vi "sub_USRP_init_Rx.vi"(11 "Rx Parameters":T1={"IQ rate (Hz)"=200000.0, "Carrier frequency [Hz]"=1187500000.0, "Gain [dB]"=16.0, "Antenna"="RX1", "Rx device name"="192.168.10.4; 192.168.10.5;"} {"Gain [dB]" format="%#_6f"; "Carrier frequency [Hz]" format="%#_6p"; "IQ rate (Hz)" format="%#_6p"}) -> (0 "Error out":errorcluster, 3 "Rx Session handle out":refnum<k15>="192.168.10.3 (5)")   [LabVIEW 2012]
uses:
  <instrlib>/niUSRP/niUSRP Timestamp.ctl
  <instrlib>/niUSRP/niUSRP Configure Time Start Trigger.vi
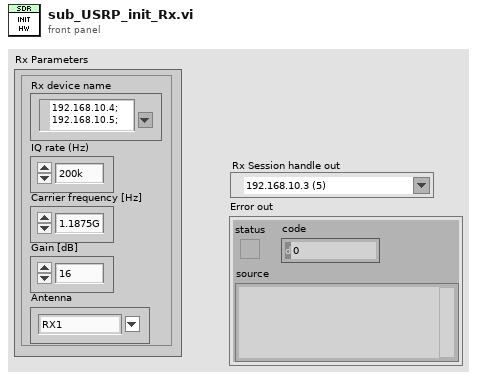
[diagram p1: front panel]
types:
  T1 = cluster{"IQ rate (Hz)":dbl, "Carrier frequency [Hz]":dbl, "Gain [dB]":dbl, "Antenna":string, "Rx device name":refnum<k15>}
  T2 = typedef "niUSRP Timestamp.ctl" = cluster{"whole seconds":u64, "fractional seconds":dbl}
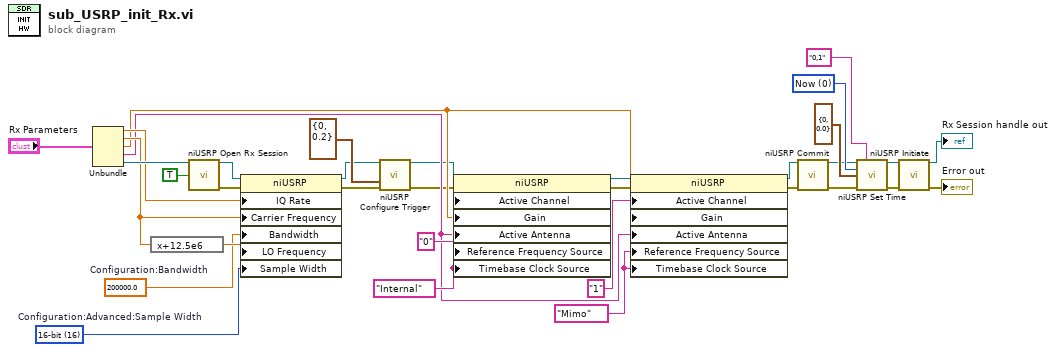
[diagram p0: block diagram]
diagram:
  w7 = 0 items=["Now", "Next Timebase Edge"] ("apply timestamp")
  w22 = "Mimo" ("Clocking and Synchronization:Reference Frequency Source")
  w20 = 200000.0  # Configuration:Bandwidth
  w19 = 16 items=["16-bit"=16, "8-bit"=8]  # Configuration:Advanced:Sample Width
  w27 = "Internal" ("Clocking and Synchronization:Reference Frequency Source")
  n1 = Unbundle("Rx Parameters") -> ("IQ rate (Hz)"=w31:dbl, "Carrier frequency [Hz]"=w30:dbl, "Gain [dB]"=w21:dbl, "Antenna"=w23:string, "Rx device name"=w33:refnum<k15>)
  n2 = expression code="x+12.5e6"(w30) -> (w29:dbl)
  n3 = call <instrlib>:"niUSRP Open Rx Session.vi"("device names"=w33, "reset"=TRUE) -> ("session handle out"=w18:refnum<k15>, "error out"=w17:errorcluster)  [unwired: 12 in]
  n4 = property class="niUSRP"(reference=w18, error in=w17, "IQ Rate"=w31, "Carrier Frequency"=w30, "Bandwidth"=w20, "LO Frequency"=w29, "Sample Width"=w19) -> (reference out=w16:refnum<k15>, error out=w15:errorcluster)
  n5 = call-poly <instrlib>:"niUSRP Configure Trigger.vi"("session handle"=w16, "start trigger time"=T2 {"whole seconds"=0, "fractional seconds"=0.2}, "error in (no error)"=w15) -> ("session handle out"=w14:refnum<k15>, "error out"=w13:errorcluster)  [unwired: 11 in]
  n6 = property class="niUSRP"(reference=w14, error in=w13, "Active Channel"="0", "Gain"=w21, "Active Antenna"=w23, "Reference Frequency Source"=w27, "Timebase Clock Source"=w27) -> (reference out=w25:refnum<k15>, error out=w24:errorcluster)
  n7 = property class="niUSRP"(reference=w25, error in=w24, "Active Channel"="1", "Gain"=w21, "Active Antenna"=w23, "Reference Frequency Source"=w22, "Timebase Clock Source"=w22) -> (reference out=w12:refnum<k15>, error out=w11:errorcluster)
  n8 = call <instrlib>:"niUSRP Commit.vi"("session handle"=w12, "error in (no error)"=w11) -> ("session handle out"=w4:refnum<k15>, "error out"=w3:errorcluster)  [unwired: 12 in]
  n9 = call <instrlib>:"niUSRP Set Time.vi"("session handle"=w4, "channel list"="0,1", "apply timestamp"=w7, "timestamp"=T2 {"whole seconds"=0, "fractional seconds"=0.0}, "error in (no error)"=w3) -> ("session handle out"=w10:refnum<k15>, "error out"=w9:errorcluster)  [unwired: 9 in]
  n10 = call <instrlib>:"niUSRP Initiate.vi"("session handle"=w10, "error in (no error)"=w9) -> ("session handle out"=→"Rx Session handle out":refnum<k15>, "error out"=→"Error out":errorcluster)  [unwired: 12 in]
